vi "Elapsed Time.vi"(11 "Start Time":u32) -> (1 "Elapsed Time":dbl)   [LabVIEW 2017]
uses:
  Global Elapsed time.vi
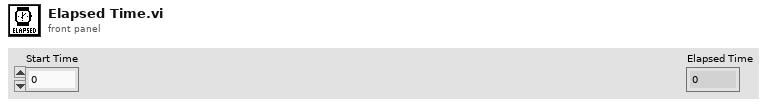
[diagram p1: front panel]
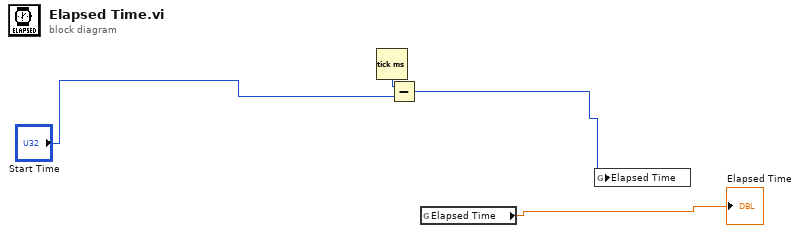
[diagram p0: block diagram]
diagram:
  n1 = Tick Count (ms)() -> (millisecond timer value=w3:u32)
  n2 = Subtract(x=w3, y="Start Time") -> (x-y=w4:u32)
  n3 = global read "Global Elapsed time.vi" "Elapsed Time"() -> (→"Elapsed Time":dbl)
  n4 = global write "Global Elapsed time.vi" "Elapsed Time"(w4) -> ()
